vi "clear board.vi"(8 "error in (no error)":errorcluster, 10 "Board":u16, 11 "identifier":string) -> (0 "error out":errorcluster, 3 "function return":bool)   [LabVIEW 2015, in "XGL_DPP.lvlib"]
doc: "EXTERN DECLSPEC bool CALL_CONV clear_board(const char* identifier, unsigned short Board);"
uses:
  XGL_DPP.lvlib
  D:/Scanning Software_Demokritos_2015_v6/libs/XGL_DPP.dll
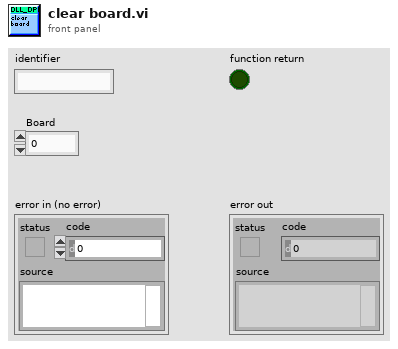
[diagram p1: front panel]
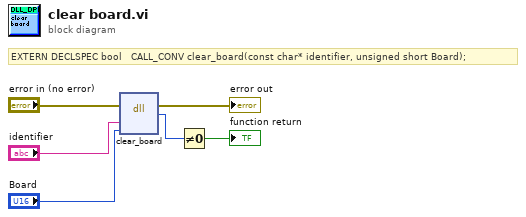
[diagram p0: block diagram]
diagram:
  # "EXTERN DECLSPEC bool   CALL_CONV clear_board(const char* identifier, unsigned short Board);"
  n1 = dll-call lib="D:/Scanning Software_Demokritos_2015_v6/libs/XGL_DPP.*" fn="clear_board"(error in="error in (no error)", "identifier"="identifier", "Board"="Board") -> (error out=→"error out":errorcluster, "return type"=w5:u8)  [unwired: 4 in, 1 out]
  n2 = Not Equal To 0?(x=w5) -> (x != 0?=→"function return":bool)
